vi "send arr of some type.vi"() -> ()   [LabVIEW 2018, in "LV2Julia_core.lvlib"]
uses:
  LV2Julia_core.lvlib
  VIs/Commands.ctl
  example server response cluster.ctl
  VIs/commands LV2Jl.ctl
  cb7a600e-1a3f-45a0-9149-1773accb9ab7.vi
  VIs/Server or client state.ctl
  5d385633-7562-4640-8300-e9530f023818.vi
  9ad41121-06aa-4420-b411-b77d699816f6.vi
  VIs/Bindata description.ctl
  VIs/bindata-only cluster.ctl
  Julia functions enum.ctl
  c1ad7611-f00e-47ba-b950-502655f00f75.vi
  <vilib>/addons/zeromq/zmq_socket.lvclass
  example args cluster.ctl
panel:
  out "element":sgl
  in  "index to return":cluster{"idx":u16[]}={"idx"=[1, 1, 1]} {"idx" min=1}
  out "appended array":sgl[][][](array[numeric])
  in  "stop LV only":bool
  out "JSON args":string
  out "LV Client state out":T1
  out "Jl Server state out":T1
  out "size(s)":i32
  out "unsigned byte array":u8[](array[numeric])
  out "short err code":u8
  out "parsed response 2":cluster{"nums":dbl[]}
  in  "go once":bool
  out "JSON out":string
  out "parsed response":T2 {"bin_lng" format="%.0e"}
  out "final error":errorcluster
  out "current error":errorcluster
  out "status":string
  in  "stop":bool
  in  "Arguments":T3={"arg1"=1, "arg2"=3.14}
  in  "fun2call":T4
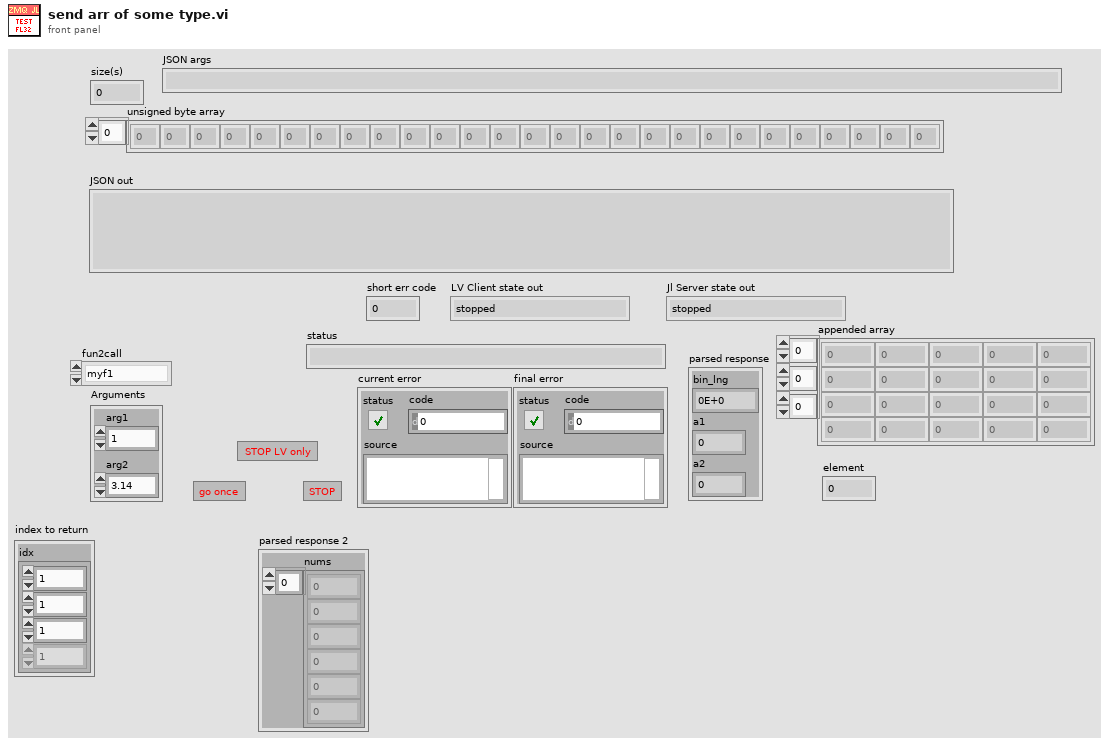
[diagram p1: front panel]
types:
  T1 = typedef "LV2Julia_core.lvlib/Server or client state.ctl" = enum16{"stopped", "running", "unknown"}
  T2 = typedef "LV-0mq-Julia_roundtrip-lib.lvlib/example server response cluster.ctl" = cluster{"bin_lng":i32, "a1":i32, "a2":dbl}
  T3 = typedef "LV-0mq-Julia_roundtrip-lib.lvlib/example args cluster.ctl" = cluster{"arg1":i32, "arg2":dbl}
  T4 = typedef "Julia functions enum.ctl" = enum16{"myf1", "myf2", "myf3", "test_bin2nums", "test_rgbimg", "numarr_loopback", "numarrs_lpbk", "Not_a_Fun"}
  T5 = typedef "LV2Julia_core.lvlib/Commands.ctl" = enum16{"Start Jl-server & Init LV-client", "Send request & Get response ", "Stop Jl-server & Cleanup LV-client", "Cleanup LV-client", "Start Jl-server", "Stop Jl-server", "Init LV-Client", "Cleanup LV-Client", "(not allowed)", "Set LV Client state", "Set Jl Server state", "set ZMQ timeout", "read ZMQ timeout", "read-out state"}
  T6 = typedef "LV2Julia_core.lvlib/bindata-only cluster.ctl" = cluster{"bindata_descr":T7[]}
  T7 = typedef "LV2Julia_core.lvlib/Bindata description.ctl" = cluster{"nofbytes":i32, "numtype":string, "start":i32, "arrdims":i32[], "kwarg_name":string, "category":string}
  T8 = typedef "LV2Julia_core.lvlib/commands LV2Jl.ctl" = u8
  T9 = typedef "LV2Julia_core.lvlib/Bindata&description.ctl" = cluster{"bindata_descr":T7[], "bindata":u8[]}
  T10 = typedef "LV2Julia_core.lvlib/detailed error info.ctl" = cluster{"exception_or_info":string, "trace":T11[]}
  T11 = typedef "LV2Julia_core.lvlib/StackFrame.ctl" = cluster{"frame_summary":string, "func":string, "linfo":string, "file":string, "line":i32, "pointer":u64, "from_c":bool, "inlined":bool}
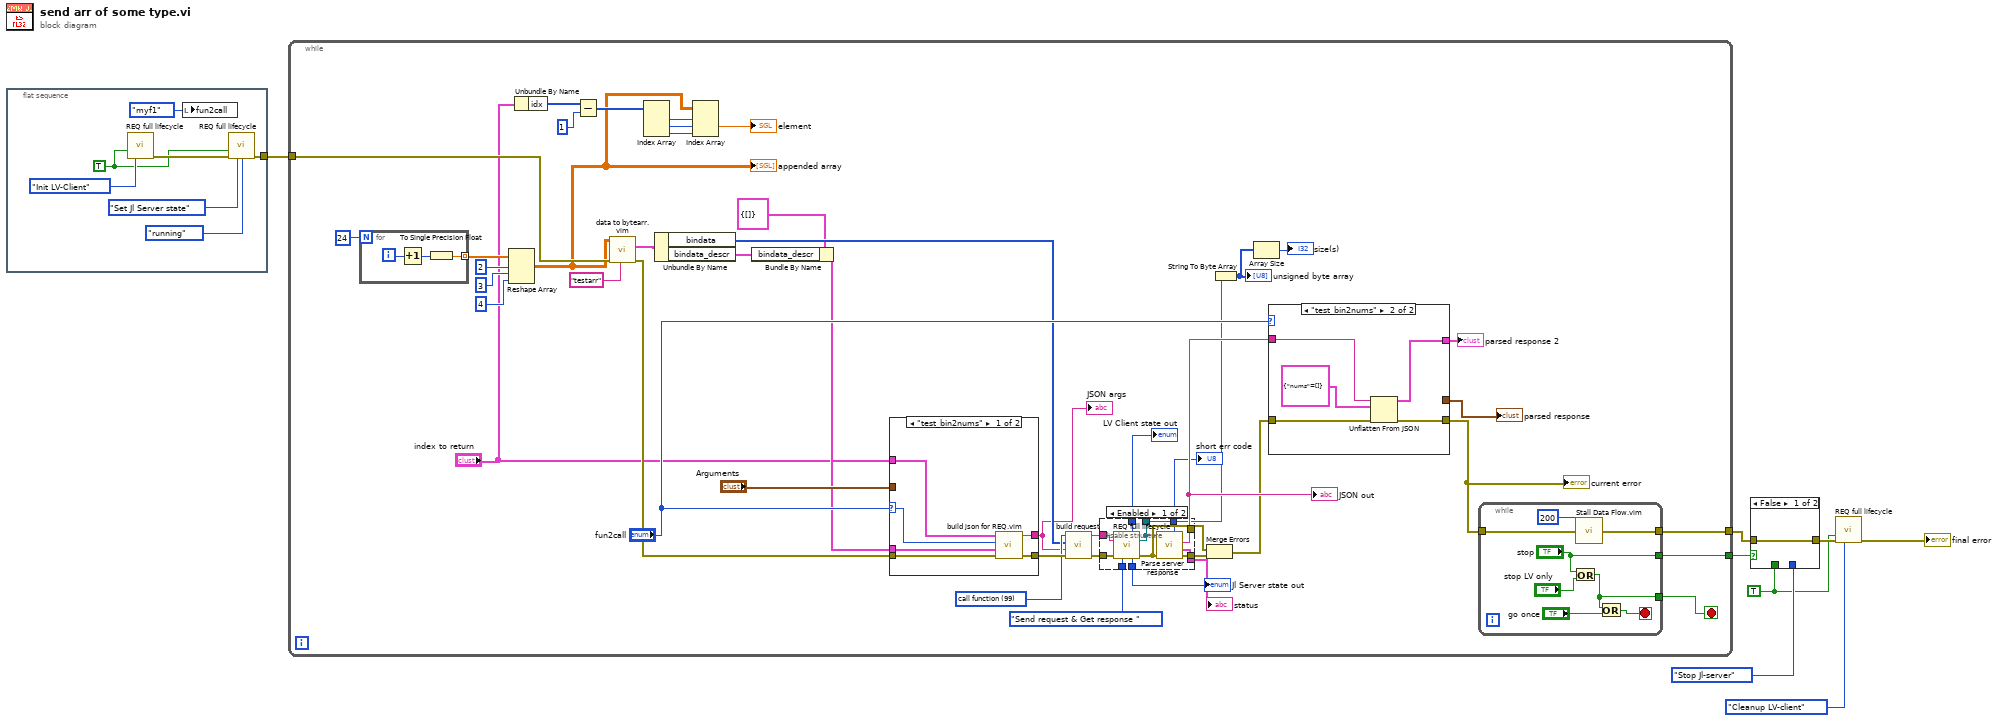
[diagram p0: block diagram]
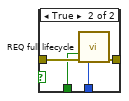
[diagram p2: hidden frame]
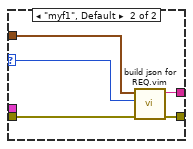
[diagram p4: hidden frame]
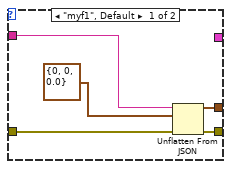
[diagram p5: hidden frame]
diagram:
  w3 = TRUE ("Force command")
  n1 = flat-sequence {
    tunnel: [w13] -> w2
    frame #0 {
      w11 = TRUE ("Force command")
      n2 = call "REQ full lifecycle.vi"("Force command"=w11, "command"=Commands."Init LV-Client") -> ("error out"=w14:errorcluster)  [unwired: 7 in, 6 out]
      n3 = local write "fun2call"(Julia_functions_enum."myf1" ("fun2call")) -> ()
      n4 = call "REQ full lifecycle.vi"("Force command"=w11, "error in"=w14, "command"=Commands."Set Jl Server state", "Jl Server state in"=Server_or_client_state."running") -> ("error out"=w13:errorcluster)  [unwired: 5 in, 6 out]
    }
  }
  n5 = while {
    tunnel: w2 -> [w32]
    tunnel: [w52] -> w8
    tunnel: [w31] -> w1
    stop <- w51 stop-if-true
    w49 = T8 99 items=["call function"=99, "ping"=112, "stop"=115] ("Command")
    n6 = for {
      N: 24 -> [_]
      tunnel: [w63] -> w28 mode=indexing
      i -> [w65]
      n7 = Increment(x=w65) -> (x+1=w64:i32)
      n8 = To Single Precision Float(number=w64) -> (single precision float=w63:sgl)
    }
    n9 = Reshape Array(w28, 2 ("dimension size"), 3 ("dimension size"), 4 ("dimension size")) -> (w20:sgl[][][])
    "appended array" <- w20
    n10 = Unbundle By Name("index to return") -> ("idx"=w23:u16[])
    n11 = Subtract(x=w23, y=1) -> (x-y=w21:i32[])
    n12 = call "data to bytearr.vim"("kwarg_name"="testarr" ("Tag"), "error in (no error)"=w32, "data in"=w20) -> ("error out"=w45:errorcluster, "Bindata & descr out"=w44:T9)  [unwired: 6 in, 1 out]
    n13 = Index Array(array=w21) -> (element #1=w19:i32, element #2=w18:i32, element #3=w17:i32)  [unwired: 3 in]
    n14 = Unbundle By Name(w44) -> ("bindata"=w42:u8[], "bindata_descr"=w34:T7[])
    n15 = Index Array(array=w20, index (dim 0)=w19, index (dim 1)=w18, index (dim 2)=w17) -> (element=→"element":sgl)
    n16 = Bundle By Name(cluster=T6 {"bindata_descr"=[]} ("bindata_only"), "bindata_descr"=w34) -> (w33:T6)
    n17 = case shown="\"test_bin2nums\"" "fun2call" {
      selector: "fun2call" -> [w79 w84]
      tunnel: [w81 w86] -> w59
      tunnel: [w80 w85] -> w30
      tunnel: w45 -> [w82 w87]
      tunnel: w33 -> [w78 _]
      tunnel: "Arguments" -> [_ w83]
      tunnel: "index to return" -> [w77 _]
      frame "test_bin2nums" {
        n18 = call "build json for REQ.vim"("error in (no error)"=w82, 9:w78, "Arguments 2"=w79, "Arguments 1"=w77) -> ("error out"=w81:errorcluster, "JSON string out"=w80:string)  [unwired: 5 in, 1 out]
      }
      frame "myf1", Default {
        n19 = call "build json for REQ.vim"("error in (no error)"=w87, "Arguments 2"=w84, "Arguments 1"=w83) -> ("error out"=w86:errorcluster, "JSON string out"=w85:string)  [unwired: 6 in, 1 out]
      }
    }
    "JSON args" <- w30
    n20 = call "build request.vi"("error in (no error)"=w59, "JSON data"=w30, "binary data"=w42, "Command"=w49) -> ("error out"=w57:errorcluster, "REQ string"=w58:string)  [unwired: 6 in]
    n21 = disable-structure shown="Enabled" {
      disable-tunnel: [w76 _] -> w62
      disable-tunnel: [w75 _] -> w61
      disable-tunnel: w58 -> [w74 _]
      disable-tunnel: w57 -> [w73 _]
      disable-tunnel: [w72 _] -> w56
      disable-tunnel: [w71 _] -> w55
      disable-tunnel: Commands."Send request & Get response " ("command") -> [w70 _]
      disable-tunnel: [w69 _] -> w41
      disable-tunnel: [w68 _] -> w40
      disable-tunnel: [w67 _] -> w37
      disable-tunnel: [w66 _] -> w36
      frame Enabled {
        n22 = call "REQ full lifecycle.vi"("data to send"=w74, "error in"=w73, "command"=w70) -> ("LV Client state out"=w66:T1, "socket out"=w68:refnum<class "zmq_socket.lvclass">, "Jl Server state out"=w67:T1, "error out"=w71:errorcluster)  [unwired: 6 in, 3 out]
        n23 = call "Parse server response.vi"("error in (no error)"=w71, "server response in"=w68) -> ("error out"=w72:errorcluster, "detailed error info"=w76:T10, "JSON out"=w75:string, "return code"=w69:u8)  [unwired: 2 in, 4 out]
      }
      frame Disabled {
      }
    }
    "status" <- w62
    "JSON out" <- w61
    "short err code" <- w41
    "Jl Server state out" <- w37
    "LV Client state out" <- w36
    n24 = Merge Errors(w55, w56) -> (w60:errorcluster)
    n25 = String To Byte Array(string=w40) -> (unsigned byte array=w39:u8[])
    "unsigned byte array" <- w39
    n26 = Array Size(array=w39) -> (size(s)=→"size(s)":i32)
    n27 = case shown="\"test_bin2nums\"" "fun2call" {
      tunnel: w61 -> [w100 w105]
      tunnel: w60 -> [w99 w104]
      tunnel: [w98 w103] -> w53
      tunnel: [w97 _] -> w50
      tunnel: [_ w101] -> w48
      frame "myf1", Default {
        n28 = Unflatten From JSON(JSON string=w100, type and defaults=T2 {"bin_lng"=0, "a1"=0, "a2"=0.0} ("parsed response"), error in (no error)=w99) -> (value=w97:T2, error out=w98:errorcluster)  [unwired: 4 in]
      }
      frame "test_bin2nums" {
        n29 = Unflatten From JSON(JSON string=w105, type and defaults=cluster{"nums":dbl[]} {"nums"=[]} ("parsed response"), error in (no error)=w104) -> (value=w101:cluster{"nums":dbl[]}, error out=w103:errorcluster)  [unwired: 4 in]
      }
    }
    "current error" <- w53
    "parsed response" <- w50
    "parsed response 2" <- w48
    n30 = while {
      tunnel: w53 -> [w95]
      tunnel: [w94] -> w52
      tunnel: [w90] -> w51
      tunnel: ["stop"] -> w31
      stop <- w91 stop-if-true
      n31 = Or(x="stop", y="stop LV only") -> (x .or. y?=w90:bool)
      n32 = call "Stall Data Flow.vim"("value in"=w95, "milliseconds to wait"=u32 200) -> ("value out"=w94:errorcluster)  [unwired: 1 out]
      n33 = Or(x=w90, y="go once") -> (x .or. y?=w91:bool)
    }
  }
  n34 = case shown="False" w1 {
    tunnel: w8 -> [w106 w110]
    tunnel: Commands."Stop Jl-server" ("command") -> [_ w109]
    tunnel: [w106 w108] -> w6
    tunnel: w3 -> [_ w107]
    frame False {
    }
    frame True {
      n35 = call "REQ full lifecycle.vi"("Force command"=w107, "error in"=w110, "command"=w109) -> ("error out"=w108:errorcluster)  [unwired: 6 in, 6 out]
    }
  }
  n36 = call "REQ full lifecycle.vi"("Force command"=w3, "error in"=w6, "command"=Commands."Cleanup LV-client") -> ("error out"=→"final error":errorcluster)  [unwired: 6 in, 6 out]
